vi "DWF FGEN Initialize.vi"(0 "Device Name":string, 5 "Reset":bool=TRUE caption="Reset (True)", 7 "Channel":string, 11 "Error In":errorcluster caption="Error In (no error)") -> (4 "Instrument Handle Out":u32, 15 "Error Out":errorcluster)   [LabVIEW 2015, in "DigilentWF.lvlib"]
doc: "Establishes communication with the device. This VI should be called once per session."
uses:
  <vilib>/DigilentWF/DigilentWF.lvlib
  dwf.dll
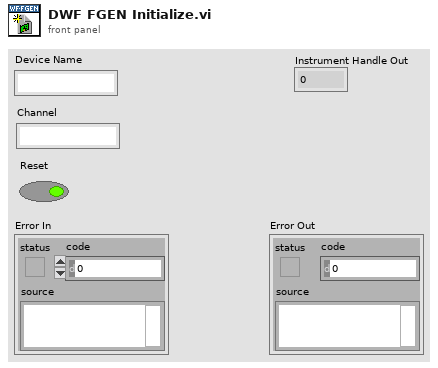
[diagram p1: front panel]
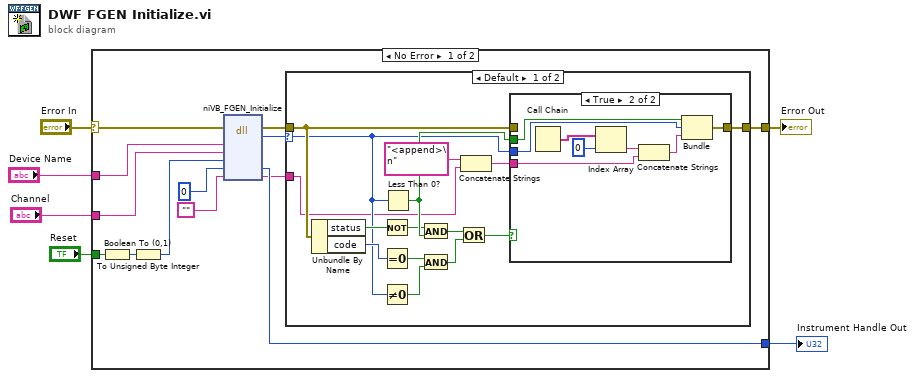
[diagram p0: block diagram]
diagram:
  n1 = case "outter_case" shown="No Error" "Error In" {
    selector: "Error In" -> [w16 w45]
    tunnel: [w19 w45] -> w5
    tunnel: "Device Name" -> [w14 _]
    tunnel: "Reset" -> [w17 _]
    tunnel: [w11 _] -> w2
    tunnel: "Channel" -> [w7 _]
    frame No Error {
      n2 = Boolean To (0,1)(Boolean=w17) -> (0, 1=w18:i16)
      n3 = To Unsigned Byte Integer(number=w18) -> (unsigned 8bit integer=w13:u8)
      n4 = dll-call lib="dwf.*" fn="niVB_FGEN_Initialize"(error in=w16, "deviceName"=w14, "channel"=w7, "reset"=w13, "instrumentHandle"=u32 0, "szError"="") -> (error out=w15:errorcluster, "return type"=w12:i32, "instrumentHandle"=w11:u32, "szError"=w9:string)  [unwired: 5 in, 1 out]
      n5 = case "inner_case" shown="Default" w12 {
        selector: w12 -> [w24 _]
        tunnel: w15 -> [w25 w44]
        tunnel: [w21 w44] -> w19
        tunnel: w9 -> [w20 _]
        frame Default {
          n6 = Unbundle By Name(w25) -> ("status"=w29:bool, "code"=w33:i32)
          n7 = Not(x=w29) -> (.not. x?=w32:bool)
          n8 = Equal To 0?(x=w33) -> (x = 0?=w28:bool)
          n9 = Not Equal To 0?(x=w24) -> (x != 0?=w31:bool)
          n10 = Less Than 0?(x=w24) -> (x < 0?=w34:bool)
          n11 = And(x=w32, y=w34) -> (x .and. y?=w30:bool)
          n12 = And(x=w28, y=w31) -> (x .and. y?=w27:bool)
          n13 = Or(x=w30, y=w27) -> (x .or. y?=w26:bool)
          n14 = Concatenate Strings("<append>\n" ("string"), w20) -> (w23:string)
          n15 = case shown="True" w26 {
            tunnel: [w35 w42] -> w21
            tunnel: w24 -> [_ w41]
            tunnel: w34 -> [_ w40]
            tunnel: w25 -> [w35 _]
            tunnel: w23 -> [_ w36]
            frame False {
            }
            frame True {
              n16 = Call Chain() -> (call chain=w39:string[])
              n17 = Index Array(array=w39, index=0) -> (element=w38:string)
              n18 = Concatenate Strings(w38, w36) -> (w43:string)
              n19 = Bundle(w40, "return type"=w41, w43) -> (w42:cluster{bool, "return type":i32, string})  [unwired: 1 out]
            }
          }
        }
        frame 0 {
        }
      }
    }
    frame Error {
    }
  }
  "Error Out" <- w5
  "Instrument Handle Out" <- w2
